vi "updateDisplay.vi"(8 "error in (no error)":errorcluster, 9 "Display Colors":cluster{"length":u32, "Color":u32}[](array[cluster]), 10 "Log Display Updated":string, 11 "reference":refnum<vi>) -> (0 "error out":errorcluster)   [LabVIEW 2017, in "Error Log.lvlib" / "Handler.UserEvent.Console.lvclass"]
uses:
  Handler.UserEvent.Console.lvclass
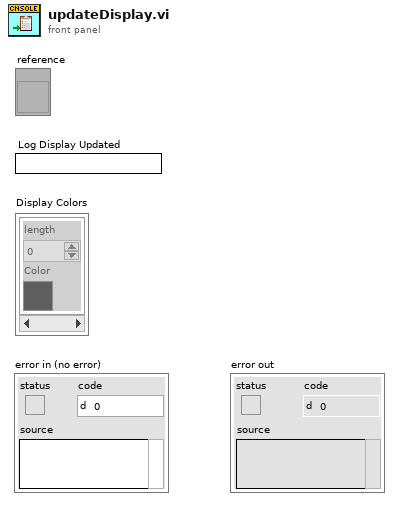
[diagram p1: front panel]
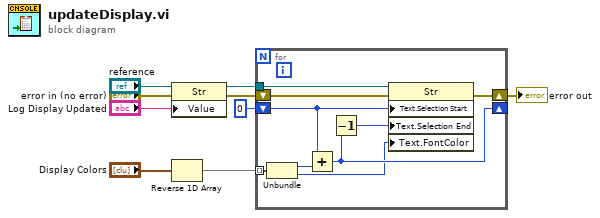
[diagram p0: block diagram]
diagram:
  n1 = property class="Str"(reference="reference", error in="error in (no error)", "Value"="Log Display Updated") -> (reference out=w6:refnum<vi>, error out=w4:errorcluster)
  n2 = Reverse 1D Array(array="Display Colors") -> (reversed array=w9:cluster{"length":u32, "Color":u32}[])
  n3 = for {
    tunnel: w9 -> [w17] mode=indexing
    tunnel: w6 -> [w18]
    shift-right: [w15] -> _
    shift-left: u32 0 -> [w16]
    shift-right: [w12] -> w2
    shift-left: w4 -> [w13]
    n4 = Unbundle(w17) -> ("length"=w11:u32, "Color"=w10:u32)
    n5 = Add(x=w16, y=w11) -> (x+y=w15:u32)
    n6 = Decrement(x=w15) -> (x-1=w14:u32)
    n7 = property on="Property Node" class="Str"(reference=w18, error in=w13, "Text.Selection Start"=w16, "Text.Selection End"=w14, "Text.FontColor"=w10) -> (error out=w12:errorcluster)  [unwired: 1 out]
  }
  "error out" <- w2
